vi "SetControlPars.vi"(8 "error in (no error)":errorcluster, 11 "DelayLineLS4 in":refnum<class "DLLS4.lvclass">) -> (0 "error out":errorcluster, 3 "DelayLineLS4 out":refnum<class "DLLS4.lvclass">)   [LabVIEW 2020, in "DLLS4.lvclass"]
uses:
  DLLS4.lvclass
  C:/dev/TRANCON/Classes/Delay Line/DelayLine.lvclass
  DelayLine.lvclass/DelayLine.ctl
  <vilib>/Utility/error.llb/DialogType.ctl
  <vilib>/ErrorRing/Error Ring.xnode
  DelayLine.lvclass
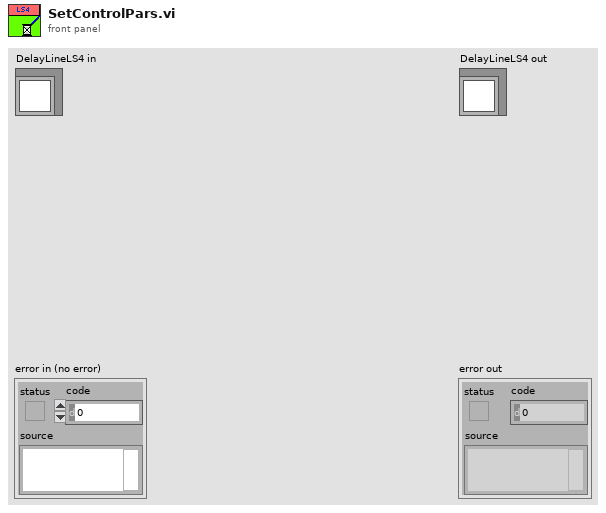
[diagram p1: front panel]
types:
  T1 = typedef "DialogType.ctl" = u16
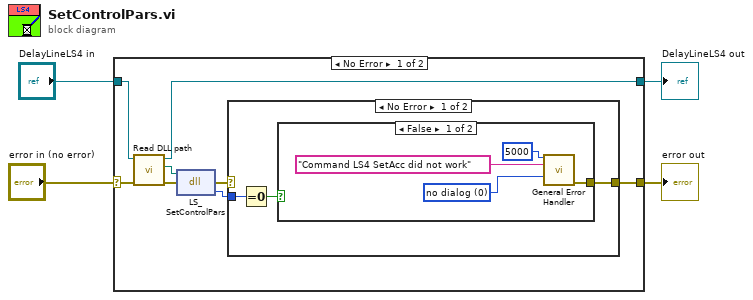
[diagram p0: block diagram]
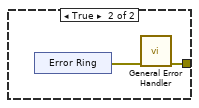
[diagram p2: hidden frame]
diagram:
  n1 = case shown="No Error" "error in (no error)" {
    selector: "error in (no error)" -> [w9 w25]
    tunnel: [w10 w25] -> w3
    tunnel: [w5 w24] -> w1
    tunnel: "DelayLineLS4 in" -> [w6 w24]
    frame No Error {
      n2 = call "Read DLL path.vi"("error in (no error)"=w9, "DelayLine in"=w6) -> ("error out"=w8:errorcluster, "DLL path"=w7:path, "DelayLine out"=w5:refnum<class "DLLS4.lvclass">)  [unwired: 7 in]
      n3 = dll-call lib="S:/TRANCON/DLL/LStep4.dll" fn="LS_SetControlPars"(path in=w7, error in=w8) -> (error out=w12:errorcluster, "type de retour"=w11:i32)  [unwired: 1 in, 1 out]
      n4 = case shown="No Error" w12 {
        selector: w12 -> [_ w23]
        tunnel: w11 -> [w15 _]
        tunnel: [w13 w23] -> w10
        frame No Error {
          n5 = Equal To 0?(x=w15) -> (x = 0?=w14:bool)
          n6 = case shown="False" w14 {
            tunnel: [w17 w20] -> w13
            frame False {
              w16 = T1 0 items=["no dialog", "OK message", "continue or stop message", "OK message + warnings", "continue/stop + warnings"] ("type of dialog (OK msg:1)")
              n7 = call <vilib>:"General Error Handler.vi"("[error code] (0)"=5000 ("code"), "[error source] (\" \")"="Command LS4 SetAcc did not work" ("String to Prepend to source (\"\")"), "type of dialog (OK msg:1)"=w16) -> ("error out"=w17:errorcluster)  [unwired: 8 in, 4 out]
            }
            frame True {
              n8 = xnode "Error Ring"() -> ("error out"=w21:errorcluster)
              n9 = call <vilib>:"General Error Handler.vi"("error in (no error)"=w21) -> ("error out"=w20:errorcluster)  [unwired: 10 in, 4 out]
            }
          }
        }
        frame Error {
        }
      }
    }
    frame Error {
    }
  }
  "error out" <- w3
  "DelayLineLS4 out" <- w1
